vi "bmptest.vi"() -> ()   [LabVIEW 2018]
uses:
  <vilib>/picture/picture.llb/imagedata.ctl
panel:
  out "size(s)":i32
  out "new picture 2":picture
  out "image data 2":T1
  out "new picture":picture
  out "image data":T1
  in  "path to BMP file":path
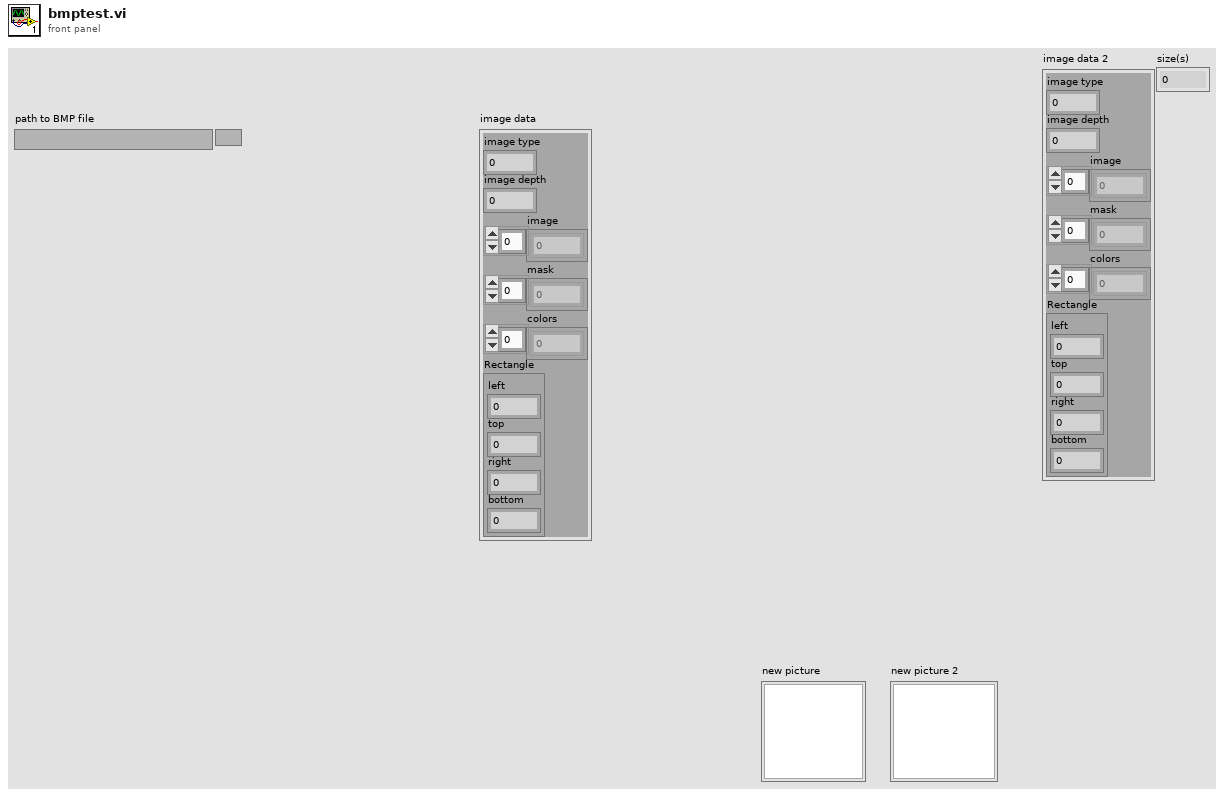
[diagram p1: front panel]
types:
  T1 = typedef "imagedata.ctl" = cluster{"image type":i32, "image depth":i32, "image":u8[], "mask":u8[], "colors":u32[], "Rectangle":cluster{"left":i16, "top":i16, "right":i16, "bottom":i16}}
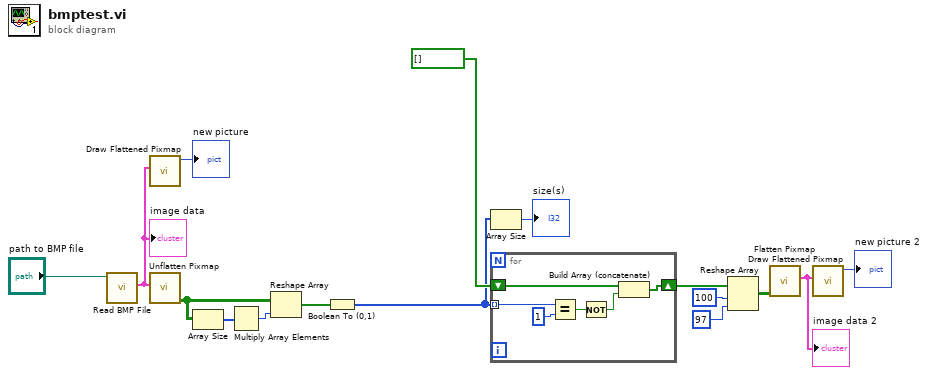
[diagram p0: block diagram]
diagram:
  n1 = call <vilib>:"Read BMP File.vi"("path to BMP file"="path to BMP file") -> ("image data"=w7:T1)  [unwired: 8 in, 2 out]
  "image data" <- w7
  n2 = call <vilib>:"Draw Flattened Pixmap.vi"("image data"=w7) -> ("new picture"=→"new picture":picture)  [unwired: 8 in]
  n3 = call <vilib>:"Unflatten Pixmap.vi"("image data"=w7) -> ("1-bit pixmap"=w5:bool[][])  [unwired: 4 in, 6 out]
  n4 = Array Size(array=w5) -> (size(s)=w6:i32[])
  n5 = Multiply Array Elements(1:w6) -> (0:w4:i32)
  n6 = Reshape Array(w5, w4) -> (w3:bool[])
  n7 = Boolean To (0,1)(Boolean=w3) -> (0, 1=w2:i16[])
  n8 = Array Size(array=w2) -> (size(s)=→"size(s)":i32)
  n9 = for {
    tunnel: w2 -> [w22] mode=indexing
    shift-right: [w20] -> w8
    shift-left: bool[] [] -> [w19]
    n10 = Equal?(x=w22, y=1) -> (x = y?=w18:bool)
    n11 = Not(x=w18) -> (.not. x?=w17:bool)
    n12 = Build Array (concatenate)(w19, w17) -> (w20:bool[])
  }
  n13 = Reshape Array(w8, 100 ("dimension size"), 97 ("dimension size")) -> (w11:bool[][])
  n14 = call <vilib>:"Flatten Pixmap.vi"("1-bit pixmap"=w11) -> ("image data"=w10:T1)  [unwired: 10 in]
  "image data 2" <- w10
  n15 = call <vilib>:"Draw Flattened Pixmap.vi"("image data"=w10) -> ("new picture"=→"new picture 2":picture)  [unwired: 8 in]
